vi "Write Target.vi"(8 "error in (no error)":errorcluster, 10 "target":dbl[unit] caption="Target", 11 "Power Supply in":refnum<class "Power Supply.lvclass">) -> (0 "error out":errorcluster, 3 "Power Supply out":refnum<class "Power Supply.lvclass">)   [LabVIEW 2009, in "Power Supply.lvclass"]
uses:
  Power Supply.lvclass
  Power Supply.lvclass/Power Supply.ctl
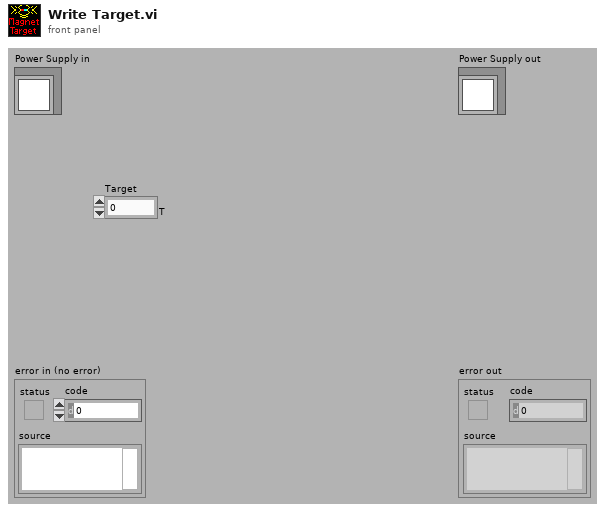
[diagram p1: front panel]
types:
  T1 = typedef "PSIO.ctl" = cluster{"Address":T2, "Version":enum16{"PS", "IPS"}}
  T2 = typedef "OxfordAddress.ctl" = cluster{"Com Port":i32, "ISOBUS Address":i32, "GPIB Address":i16, "Communication":enum16{"RS232", "ISOBUS", "GPIB", "Gateway"}}
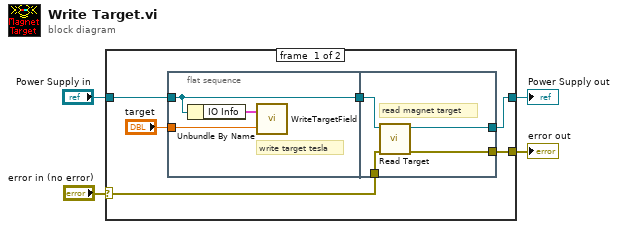
[diagram p0: block diagram]
diagram:
  n1 = case shown="No Error" "error in (no error)" {
    selector: "error in (no error)" -> [w7 w18]
    tunnel: "Power Supply in" -> [w6 w19]
    tunnel: [w9 w19] -> w2
    tunnel: [w8 w18] -> w1
    frame #0 {
      n2 = flat-sequence {
        tunnel: "target" -> [w11]
        tunnel: w6 -> [w13]
        tunnel: [w13] -> w5
        tunnel: [w17] -> w9
        tunnel: [w16] -> w8
        tunnel: w7 -> [w15]
        tunnel: w5 -> [w14]
        frame #0 {
          # "write target tesla"
          n3 = Unbundle By Name(w13) -> ("IO Info"=w12:T1)
          n4 = call "WriteTargetField.vi"("Target Field"=w11, "IO Info"=w12) -> ()  [unwired: 2 out]
        }
        frame #1 {
          # "read magnet target"
          n5 = call-dynamic "Read Target.vi"("error in (no error)"=w15, "Power Supply in"=w14) -> ("error out"=w16:errorcluster, "Power Supply out"=w17:refnum<class "Power Supply.lvclass">)  [unwired: 7 in, 1 out]
        }
      }
    }
    frame #1 {
    }
  }
  "error out" <- w1
  "Power Supply out" <- w2
